vi "Rising-Falling Edge Midpoints.vi"(5 "High Level":dbl, 7 "Low Level":dbl, 8 "Error In":errorcluster, 11 "Amplitude array":dbl[](array[numeric])) -> (0 "Error Out":errorcluster, 1 "Falling Edge Midpoint Index":dbl, 2 "Midpoint":dbl, 3 "Rising Edge Midpoint Index":dbl)   [LabVIEW 2021, in "Fits.lvlib"]
uses:
  Fits.lvlib
  Math/Math.lvlib
  Arrays/Arrays.lvlib
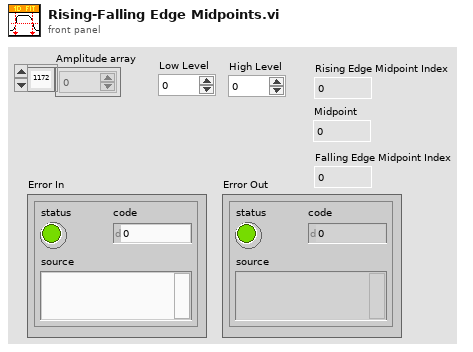
[diagram p1: front panel]
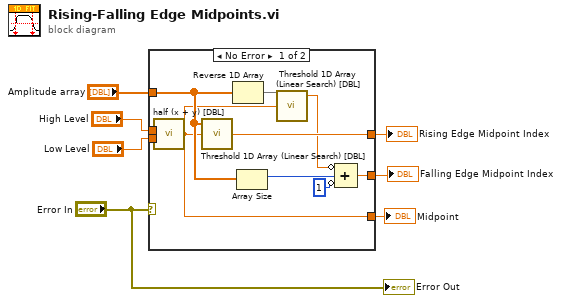
[diagram p0: block diagram]
diagram:
  n1 = case shown="No Error" "Error In" {
    tunnel: "Low Level" -> [w17 _]
    tunnel: "High Level" -> [w16 _]
    tunnel: [w15 _] -> w5
    tunnel: "Amplitude array" -> [w13 _]
    tunnel: [w10 _] -> w3
    tunnel: [w8 _] -> w1
    frame No Error {
      n2 = call "half (x + y) [DBL].vi"("y"=w17, "x"=w16) -> ("(x+y)/2"=w8:dbl)  [unwired: 4 in]
      n3 = call "Threshold 1D Array (Linear Search) [DBL].vi"("Array"=w13, "Y"=w8) -> ("fractional index"=w15:dbl)  [unwired: 7 in]
      n4 = Reverse 1D Array(array=w13) -> (reversed array=w14:dbl[])
      n5 = Array Size(array=w13) -> (size(s)=w11:i32)
      n6 = call "Threshold 1D Array (Linear Search) [DBL].vi"("Array"=w14, "Y"=w8) -> ("fractional index"=w12:dbl)  [unwired: 7 in]
      n7 = Compound Arithmetic op=ADD(invert w12, w11, invert 1 ("value")) -> (w10:dbl)
    }
    frame Error {
    }
  }
  "Rising Edge Midpoint Index" <- w5
  "Falling Edge Midpoint Index" <- w3
  "Midpoint" <- w1
  "Error Out" <- "Error In"
